vi "Retrieve API Key.vi"(8 "error in":errorcluster, 11 "Artifactory":refnum<class "Artifactory.lvclass">) -> (0 "error out":errorcluster, 2 "Authorization":T1, 3 "Artifactory out":refnum<class "Artifactory.lvclass">, 5 "found":bool)   [LabVIEW 2021, in "Artifactory.lvclass"]
uses:
  Artifactory.lvclass
  Authorization -- cluster.ctl
  auth-type -- enum.ctl
  f35bd4e4-f4d6-4a88-90d2-444e7f2c3e6f.vi
  <vilib>/Utility/error.llb/Error Cluster From Error Code.vi
  <vilib>/JDP Science/JSONtext/JSON text to Variant.vi
  <vilib>/ErrorRing/Error Ring.xnode
  <vilib>/JDP Science/JSONtext/LVClass Serializer/JSONtext LVClass Serializer.lvclass
  Artifactory.lvclass/Artifactory.ctl
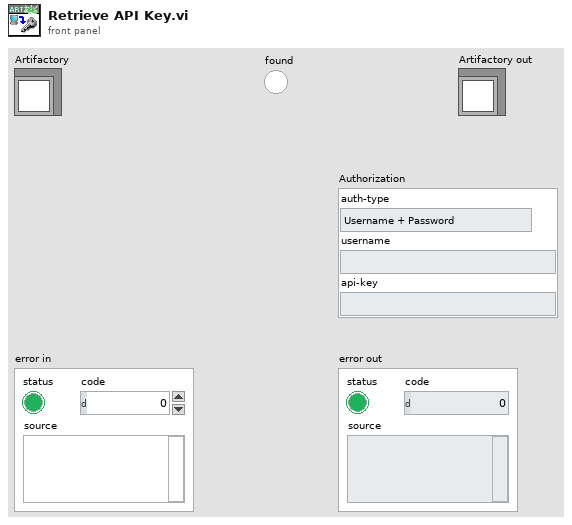
[diagram p1: front panel]
types:
  T1 = typedef "Artifactory.lvclass/Authorization -- cluster.ctl" = cluster{"auth-type":T2, "username":string, "api-key":string}
  T2 = typedef "Artifactory.lvclass/auth-type -- enum.ctl" = enum16{"Username + Password", "Username + API Key", "API Key", "Access token"}
  T3 = enum16{"open", "replace", "create", "open or create", "replace or create", "replace or create with confirmation"}
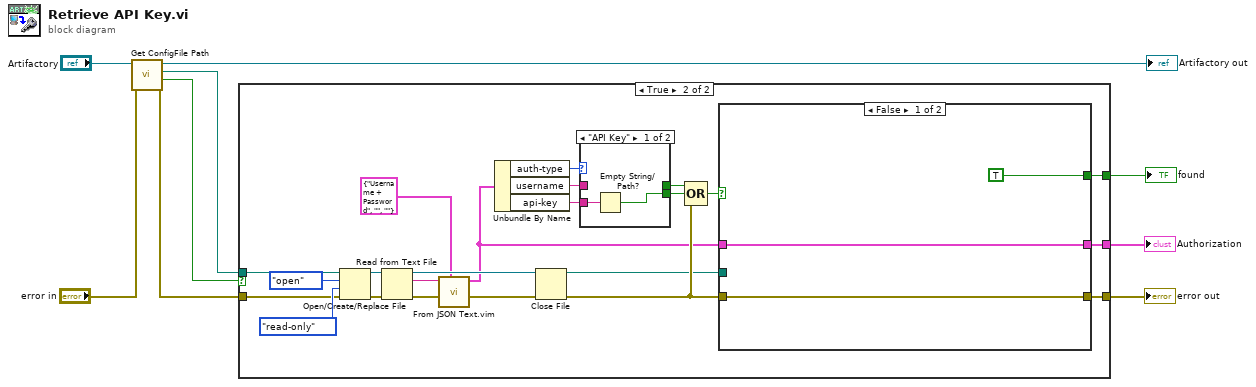
[diagram p0: block diagram]
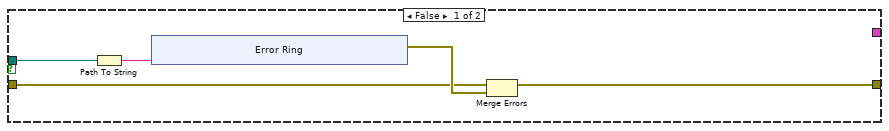
[diagram p2: hidden frame]
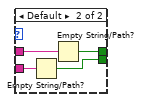
[diagram p3: hidden frame]
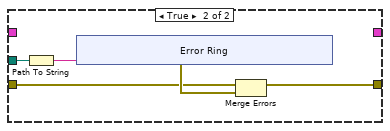
[diagram p4: hidden frame]
diagram:
  n1 = call-dynamic "Get ConfigFile Path.vi"("error in (no error)"="error in", "Artifactory in"="Artifactory") -> ("error out"=w4:errorcluster, "found"=w5:bool, "Config File"=w6:path, "Artifactory out"=→"Artifactory out":refnum<class "Artifactory.lvclass">)  [unwired: 6 in]
  n2 = case shown="True" w5 {
    tunnel: [w13 w34] -> w3
    tunnel: [_ w29] -> w2
    tunnel: w4 -> [w12 w36]
    tunnel: w6 -> [w11 w35]
    tunnel: [_ w28] -> w1
    frame False {
      n3 = Path To String(path=w11) -> (string=w10:string)
      n4 = xnode "Error Ring"("parameter 0"=w10) -> ("error out"=w14:errorcluster)
      n5 = Merge Errors(w12, w14) -> (w13:errorcluster)
    }
    frame True {
      n6 = Open/Create/Replace File(file path (use dialog)=w35, error in=w36, operation (0:open)=T3."open", access (0:read/write)=enum16{"read/write", "read-only", "write-only"}."read-only") -> (refnum out=w44:refnum<file>, error out=w42:errorcluster)  [unwired: 2 in, 1 out]
      n7 = Read from Text File(file (use dialog)=w44, error in=w42) -> (refnum out=w41:refnum<file>, text=w39:string, error out=w38:errorcluster)  [unwired: 2 in, 1 out]
      n8 = call "From JSON Text.vim"("Data Type and Default Value"=T1 {"auth-type"=enum."Username + Password", "username"="", "api-key"=""} ("Basic Authorization"), "error in (no error)"=w38, "JSON"=w39) -> ("error out"=w37:errorcluster, "Data out"=w26:T1)  [unwired: 7 in]
      n9 = Unbundle By Name(w26) -> ("auth-type"=w22:T2, "username"=w30:string, "api-key"=w31:string)
      n10 = Close File(refnum=w41, error in=w37) -> (path=w24:path, error out=w27:errorcluster)
      n11 = case shown="\"API Key\"" w22 {
        tunnel: [_ w50] -> w33
        tunnel: w31 -> [w46 w49]
        tunnel: w30 -> [_ w48]
        tunnel: [w45 w47] -> w25
        frame "API Key" {
          n12 = Empty String/Path?(string/path=w46) -> (empty?=w45:bool)
        }
        frame Default {
          n13 = Empty String/Path?(string/path=w49) -> (empty?=w47:bool)
          n14 = Empty String/Path?(string/path=w48) -> (empty?=w50:bool)
        }
      }
      n15 = Compound Arithmetic op=OR(w33, w25, w27) -> (w32:bool)
      n16 = case shown="False" w32 {
        tunnel: w27 -> [w53 w57]
        tunnel: [w53 w56] -> w34
        tunnel: [w51 _] -> w29
        tunnel: [TRUE _] -> w28
        tunnel: w26 -> [w51 _]
        tunnel: w24 -> [_ w55]
        frame False {
        }
        frame True {
          n17 = Path To String(path=w55) -> (string=w54:string)
          n18 = xnode "Error Ring"("parameter 0"=w54) -> ("error out"=w58:errorcluster)
          n19 = Merge Errors(w57, w58) -> (w56:errorcluster)
        }
      }
    }
  }
  "error out" <- w3
  "Authorization" <- w2
  "found" <- w1
